vi "generateSQL-old.vi"(1 "timestamp 2":string, 2 "timestamp":string, 3 "temp, humidity, light, co2":cluster{bool, bool, bool, bool}, 4 "mote, plc":cluster{bool, bool}) -> (0 "SQL command":string)   [LabVIEW 2011]
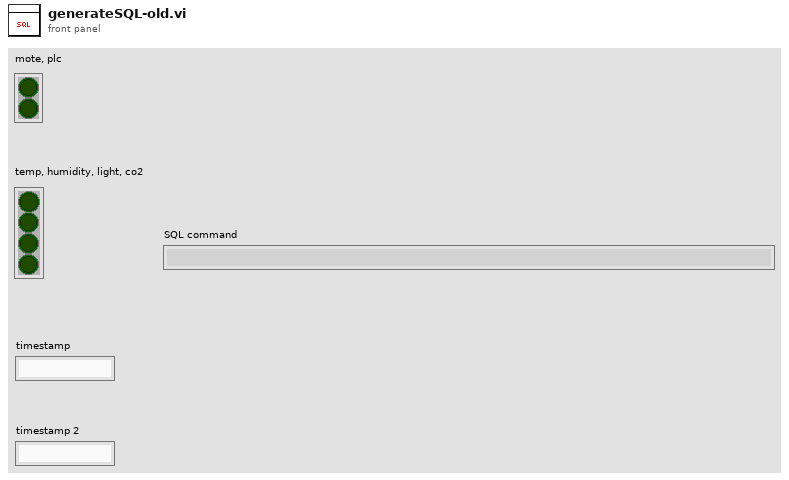
[diagram p1: front panel]
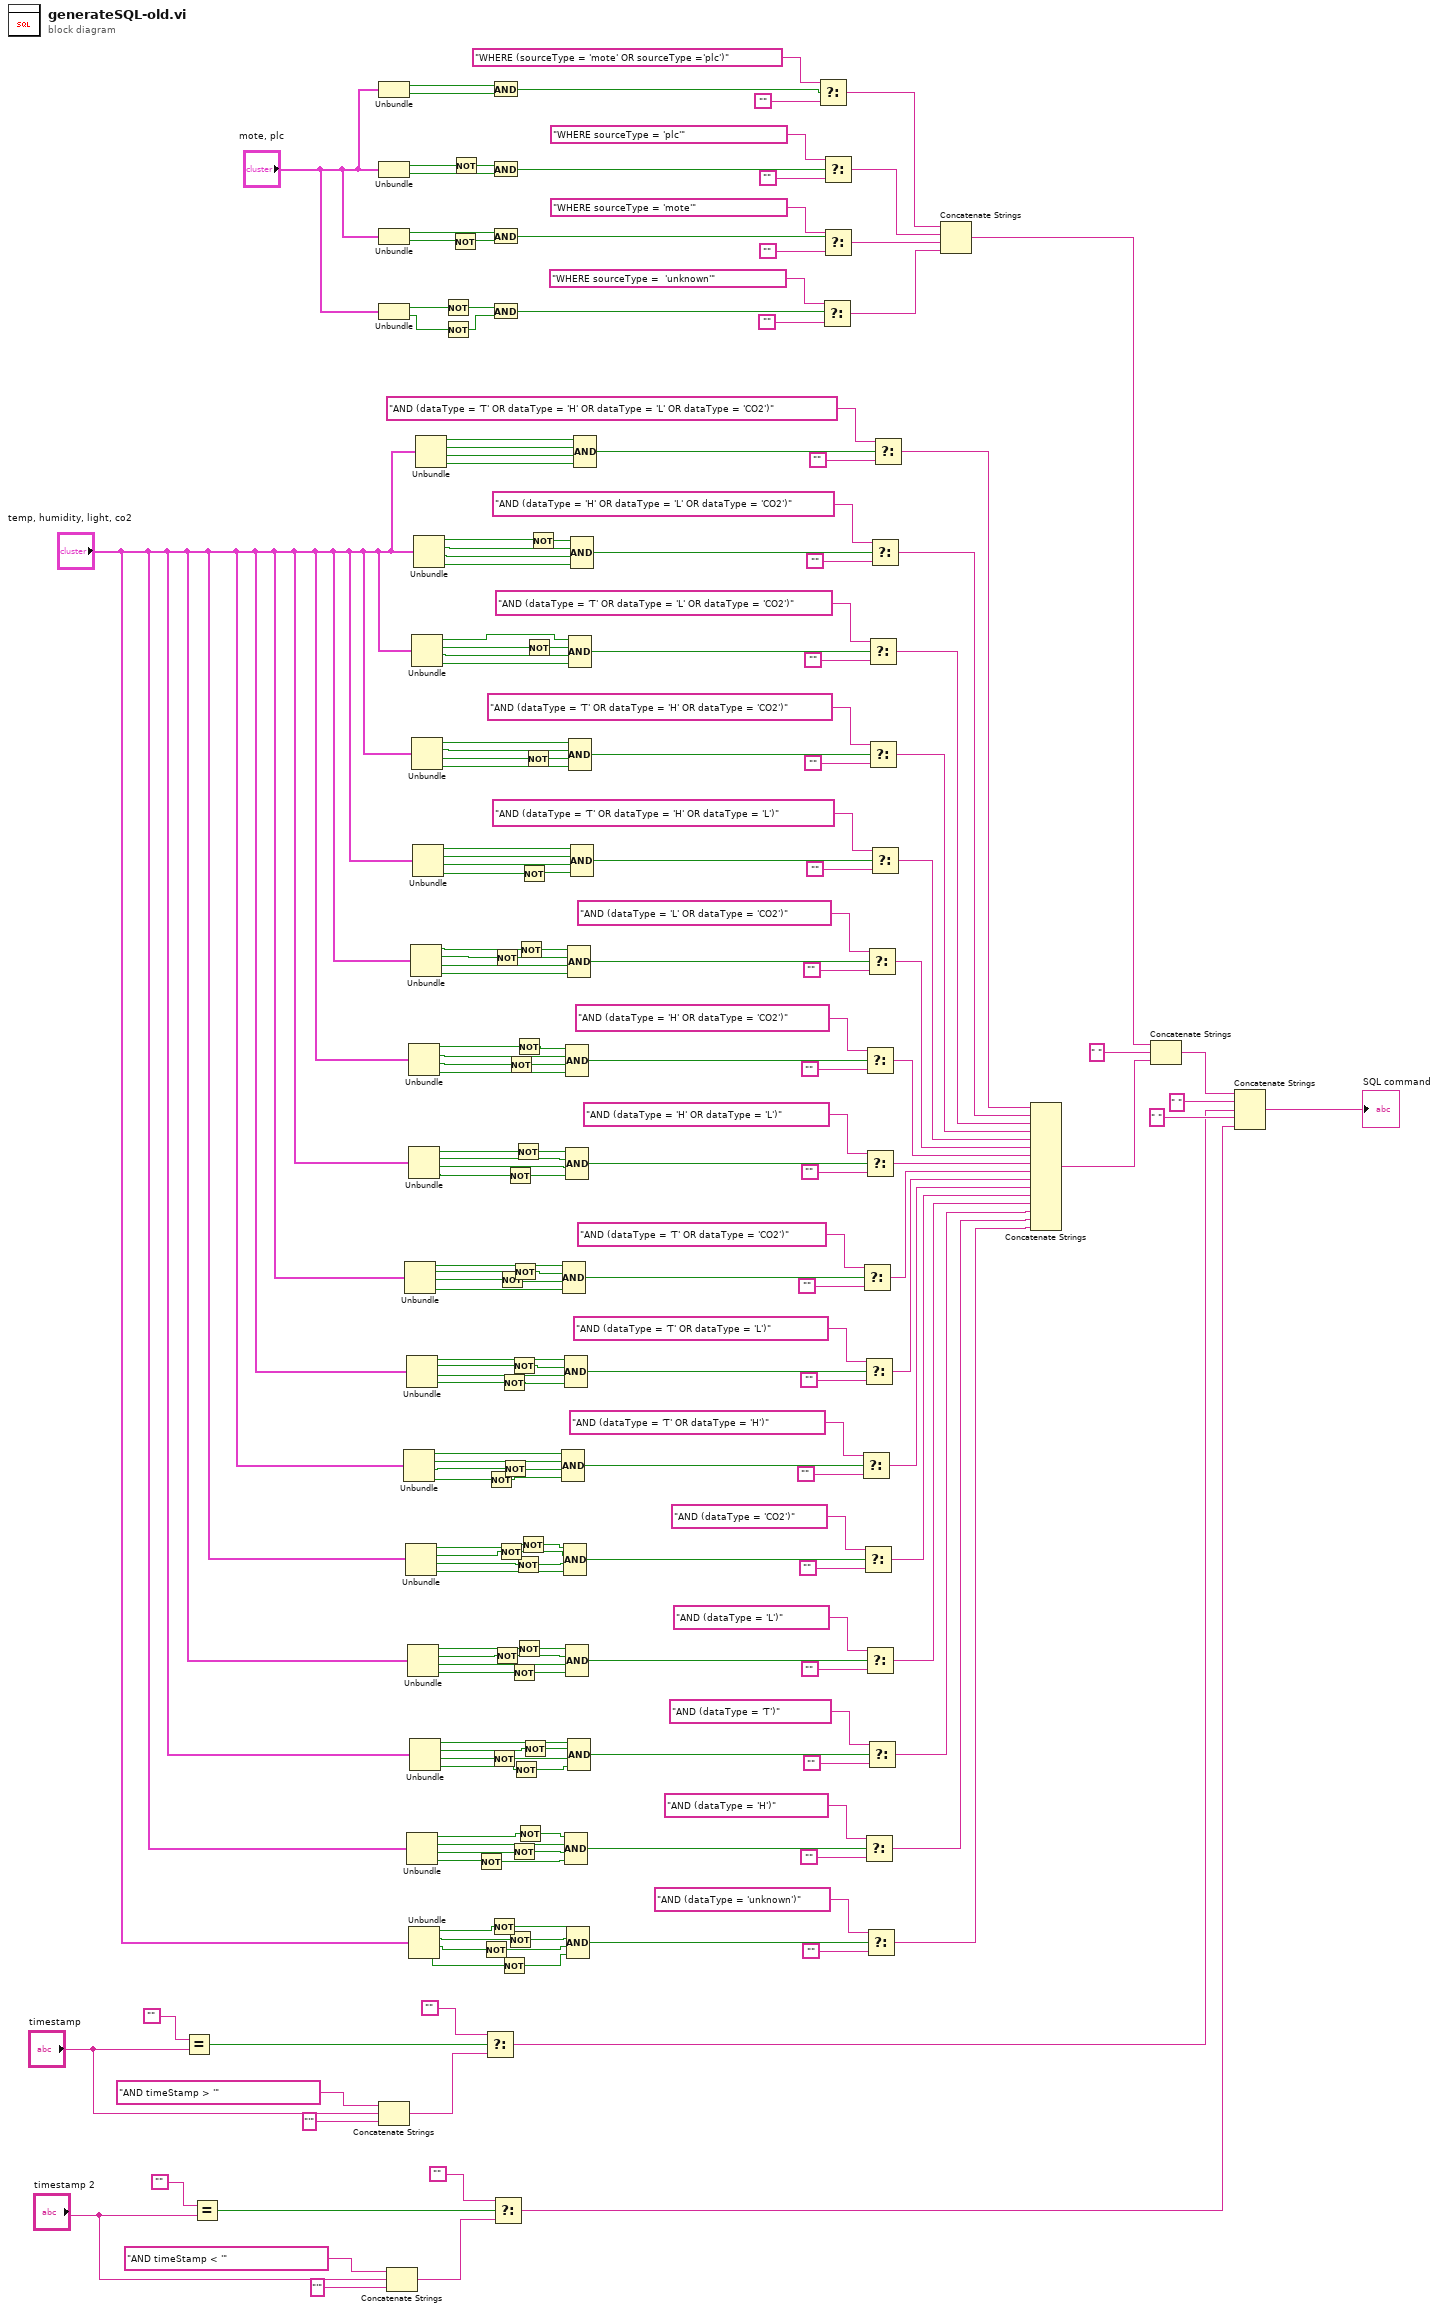
[diagram p0: block diagram]
diagram:
  n1 = Equal?(x="", y="timestamp") -> (x = y?=w15:bool)
  n2 = Equal?(x="", y="timestamp 2") -> (x = y?=w8:bool)
  n3 = Unbundle("mote, plc") -> (w190:bool, w189:bool)
  n4 = Unbundle("mote, plc") -> (w209:bool, w208:bool)
  n5 = Unbundle("mote, plc") -> (w188:bool, w187:bool)
  n6 = Unbundle("mote, plc") -> (w186:bool, w185:bool)
  n7 = Concatenate Strings("AND timeStamp > '", "timestamp", "'") -> (w12:string)
  n8 = Concatenate Strings("AND timeStamp < '", "timestamp 2", "'") -> (w10:string)
  n9 = Unbundle("temp, humidity, light, co2") -> (w86:bool, w85:bool, w83:bool, w81:bool)
  n10 = Unbundle("temp, humidity, light, co2") -> (w96:bool, w94:bool, w92:bool, w91:bool)
  n11 = Unbundle("temp, humidity, light, co2") -> (w80:bool, w78:bool, w76:bool, w74:bool)
  n12 = Unbundle("temp, humidity, light, co2") -> (w90:bool, w21:bool, w20:bool, w87:bool)
  n13 = Unbundle("temp, humidity, light, co2") -> (w59:bool, w57:bool, w56:bool, w54:bool)
  n14 = Unbundle("temp, humidity, light, co2") -> (w72:bool, w71:bool, w69:bool, w68:bool)
  n15 = Unbundle("temp, humidity, light, co2") -> (w131:bool, w130:bool, w129:bool, w127:bool)
  n16 = Unbundle("temp, humidity, light, co2") -> (w125:bool, w122:bool, w121:bool, w124:bool)
  n17 = Unbundle("temp, humidity, light, co2") -> (w52:bool, w50:bool, w48:bool, w46:bool)
  n18 = Unbundle("temp, humidity, light, co2") -> (w66:bool, w65:bool, w63:bool, w61:bool)
  n19 = Unbundle("temp, humidity, light, co2") -> (w137:bool, w135:bool, w134:bool, w133:bool)
  n20 = Unbundle("temp, humidity, light, co2") -> (w1:bool, w2:bool, w150:bool, w149:bool)
  n21 = Unbundle("temp, humidity, light, co2") -> (w148:bool, w147:bool, w145:bool, w144:bool)
  n22 = Unbundle("temp, humidity, light, co2") -> (w143:bool, w142:bool, w141:bool, w139:bool)
  n23 = Unbundle("temp, humidity, light, co2") -> (w156:bool, w154:bool, w153:bool, w152:bool)
  n24 = Unbundle("temp, humidity, light, co2") -> (w184:bool, w183:bool, w182:bool, w181:bool)
  n25 = Not(x=w186) -> (.not. x?=w211:bool)
  n26 = Not(x=w185) -> (.not. x?=w210:bool)
  n27 = Not(x=w187) -> (.not. x?=w212:bool)
  n28 = Not(x=w209) -> (.not. x?=w213:bool)
  n29 = Not(x=w54) -> (.not. x?=w53:bool)
  n30 = Not(x=w48) -> (.not. x?=w47:bool)
  n31 = Select(t="", s=w15, f=w12) -> (s? t:f=w11:string)
  n32 = Not(x=w81) -> (.not. x?=w82:bool)
  n33 = Not(x=w63) -> (.not. x?=w62:bool)
  n34 = Not(x=w52) -> (.not. x?=w51:bool)
  n35 = And(x=w190, y=w189) -> (x .and. y?=w207:bool)
  n36 = And(x=w213, y=w208) -> (x .and. y?=w198:bool)
  n37 = And(x=w188, y=w212) -> (x .and. y?=w197:bool)
  n38 = And(x=w211, y=w210) -> (x .and. y?=w196:bool)
  n39 = Not(x=w135) -> (.not. x?=w136:bool)
  n40 = Not(x=w71) -> (.not. x?=w70:bool)
  n41 = Select(t="", s=w8, f=w10) -> (s? t:f=w3:string)
  n42 = Not(x=w78) -> (.not. x?=w77:bool)
  n43 = Not(x=w92) -> (.not. x?=w93:bool)
  n44 = Not(x=w87) -> (.not. x?=w88:bool)
  n45 = Not(x=w46) -> (.not. x?=w45:bool)
  n46 = Not(x=w83) -> (.not. x?=w84:bool)
  n47 = Not(x=w124) -> (.not. x?=w123:bool)
  n48 = Not(x=w50) -> (.not. x?=w49:bool)
  n49 = Not(x=w129) -> (.not. x?=w128:bool)
  n50 = Not(x=w21) -> (.not. x?=w89:bool)
  n51 = Not(x=w68) -> (.not. x?=w67:bool)
  n52 = Not(x=w56) -> (.not. x?=w55:bool)
  n53 = Not(x=w94) -> (.not. x?=w95:bool)
  n54 = Not(x=w61) -> (.not. x?=w60:bool)
  n55 = Not(x=w125) -> (.not. x?=w126:bool)
  n56 = Not(x=w76) -> (.not. x?=w75:bool)
  n57 = Not(x=w131) -> (.not. x?=w132:bool)
  n58 = Not(x=w72) -> (.not. x?=w73:bool)
  n59 = Not(x=w59) -> (.not. x?=w58:bool)
  n60 = Not(x=w137) -> (.not. x?=w138:bool)
  n61 = Not(x=w80) -> (.not. x?=w79:bool)
  n62 = Not(x=w139) -> (.not. x?=w140:bool)
  n63 = Not(x=w65) -> (.not. x?=w64:bool)
  n64 = Not(x=w145) -> (.not. x?=w146:bool)
  n65 = Not(x=w2) -> (.not. x?=w151:bool)
  n66 = Not(x=w156) -> (.not. x?=w155:bool)
  n67 = Compound Arithmetic op=AND(w86, w85, w84, w82) -> (w111:bool)
  n68 = Compound Arithmetic op=AND(w96, w95, w93, w91) -> (w118:bool)
  n69 = Compound Arithmetic op=AND(w79, w77, w75, w74) -> (w112:bool)
  n70 = Compound Arithmetic op=AND(w90, w89, w20, w88) -> (w117:bool)
  n71 = Compound Arithmetic op=AND(w58, w57, w55, w53) -> (w106:bool)
  n72 = Compound Arithmetic op=AND(w132, w130, w128, w127) -> (w165:bool)
  n73 = Compound Arithmetic op=AND(w126, w122, w121, w123) -> (w166:bool)
  n74 = Compound Arithmetic op=AND(w73, w70, w69, w67) -> (w99:bool)
  n75 = Compound Arithmetic op=AND(w51, w49, w47, w45) -> (w105:bool)
  n76 = Compound Arithmetic op=AND(w138, w136, w134, w133) -> (w160:bool)
  n77 = Compound Arithmetic op=AND(w66, w64, w62, w60) -> (w100:bool)
  n78 = Compound Arithmetic op=AND(w1, w151, w150, w149) -> (w172:bool)
  n79 = Compound Arithmetic op=AND(w148, w147, w146, w144) -> (w171:bool)
  n80 = Compound Arithmetic op=AND(w155, w154, w153, w152) -> (w177:bool)
  n81 = Compound Arithmetic op=AND(w143, w142, w141, w140) -> (w159:bool)
  n82 = Compound Arithmetic op=AND(w184, w183, w182, w181) -> (w178:bool)
  n83 = Select(t="WHERE (sourceType = 'mote' OR sourceType ='plc')", s=w207, f="") -> (s? t:f=w195:string)
  n84 = Select(t="WHERE sourceType =  'unknown'", s=w196, f="") -> (s? t:f=w192:string)
  n85 = Select(t="WHERE sourceType = 'plc'", s=w198, f="") -> (s? t:f=w194:string)
  n86 = Select(t="WHERE sourceType = 'mote'", s=w197, f="") -> (s? t:f=w193:string)
  n87 = Select(t="AND (dataType = 'T' OR dataType = 'H')", s=w111, f="") -> (s? t:f=w33:string)
  n88 = Select(t="AND (dataType = 'T' OR dataType = 'CO2')", s=w118, f="") -> (s? t:f=w35:string)
  n89 = Select(t="AND (dataType = 'CO2')", s=w112, f="") -> (s? t:f=w32:string)
  n90 = Select(t="AND (dataType = 'T' OR dataType = 'L')", s=w117, f="") -> (s? t:f=w34:string)
  n91 = Select(t="AND (dataType = 'H')", s=w106, f="") -> (s? t:f=w29:string)
  n92 = Select(t="AND (dataType = 'H' OR dataType = 'CO2')", s=w165, f="") -> (s? t:f=w37:string)
  n93 = Select(t="AND (dataType = 'H' OR dataType = 'L')", s=w166, f="") -> (s? t:f=w36:string)
  n94 = Select(t="AND (dataType = 'L')", s=w99, f="") -> (s? t:f=w31:string)
  n95 = Select(t="AND (dataType = 'unknown')", s=w105, f="") -> (s? t:f=w28:string)
  n96 = Select(t="AND (dataType = 'L' OR dataType = 'CO2')", s=w160, f="") -> (s? t:f=w38:string)
  n97 = Select(t="AND (dataType = 'T')", s=w100, f="") -> (s? t:f=w30:string)
  n98 = Select(t="AND (dataType = 'T' OR dataType = 'L' OR dataType = 'CO2')", s=w172, f="") -> (s? t:f=w41:string)
  n99 = Select(t="AND (dataType = 'T' OR dataType = 'H' OR dataType = 'CO2')", s=w171, f="") -> (s? t:f=w40:string)
  n100 = Select(t="AND (dataType = 'H' OR dataType = 'L' OR dataType = 'CO2')", s=w177, f="") -> (s? t:f=w42:string)
  n101 = Select(t="AND (dataType = 'T' OR dataType = 'H' OR dataType = 'L')", s=w159, f="") -> (s? t:f=w39:string)
  n102 = Select(t="AND (dataType = 'T' OR dataType = 'H' OR dataType = 'L' OR dataType = 'CO2')", s=w178, f="") -> (s? t:f=w43:string)
  n103 = Concatenate Strings(w195, w194, w193, w192) -> (w27:string)
  n104 = Concatenate Strings(w43, w42, w41, w40, w39, w38, w37, w36, w35, w34, w33, w32, w31, w30, w29, w28) -> (w25:string)
  n105 = Concatenate Strings(w27, " ", w25) -> (w24:string)
  n106 = Concatenate Strings(w24, " ", w11, " ", w3) -> (→"SQL command":string)
